vi "test comm.vi"() -> ()   [LabVIEW 2010]
uses:
  <userlib>/TIO Library 2010/TIO Stream Write.vi
  <userlib>/TIO Library 2010/TIO RPC Form Request.vi
  <userlib>/TIO Library 2010/TIO SLIP Serial Write.vi
  <userlib>/TIO Library 2010/TIO Form Packet.vi
  <userlib>/TIO Library 2010/TIO SLIP Encode.vi
  <userlib>/TIO Library 2010/TIO Serial Checksum CRC32.vi
panel:
  in  "flush":bool
  in  "milliseconds to wait":u32=100
  out "appended array 2":cluster{dbl, "start":dbl, "u32":u32}[](array[cluster]) {"start" format="%#.3f"}
  in  "Enum":enum16{"straight", "dstream"}(ring)
  out "Payload at dtream":string
  out "dstream info":T1
  out "Payload at timebase":string
  out "Payload at pstream":string
  out "pstreams out":T2(array[cluster])
  out "timebases out":T3(array[cluster])
  out "Payload at type 5":string
  out "appended array":u16[](array[numeric])
  in  "TIO State":T4={"Awaiting REP"=FALSE, "REQ ID"=500, "dstreams in"=[{"id"=0, "timebase id"=1, "period"=16, "offset"=0, "sample number"=10656, "total components"=6, "flags"=1, "components"=[{"pstream id"=0, "flags"=0, "period"=1, "offset"=0}, {"pstream id"=1, "flags"=1, "period"=1, "offset"=0}, {"pstream id"=32770, "flags"=0, "period"=8, "offset"=0}, {"pstream id"=32772, "flags"=0, "period"=8, "offset"=0}, {"pstream id"=32774, "flags"=1, "period"=64, "offset"=0}, {"pstream id"=2, "flags"=1, "period"=64, "offset"=0}]}, {"id"=0, "timebase id"=0, "period"=0, "offset"=0, "sample number"=0, "total components"=0, "flags"=0, "components"=[]}, {"id"=0, "timebase id"=0, "period"=0, "offset"=0, "sample number"=0, "total components"=0, "flags"=0, "components"=[]}, {"id"=0, "timebase id"=0, "period"=0, "offset"=0, "sample number"=0, "total components"=0, "flags"=0, "components"=[]}, {"id"=0, "timebase id"=0, "period"=0, "offset"=0, "sample number"=0, "total components"=0, "flags"=0, "components"=[]}, {"id"=0, "timebase id"=0, "period"=0, "offset"=0, "sample number"=0, "total components"=0, "flags"=0, "components"=[]}, {"id"=0, "timebase id"=0, "period"=0, "offset"=0, "sample number"=0, "total components"=0, "flags"=0, "components"=[]}, {"id"=0, "timebase id"=0, "period"=0, "offset"=0, "sample number"=0, "total components"=0, "flags"=0, "components"=[]}, {"id"=0, "timebase id"=0, "period"=0, "offset"=0, "sample number"=0, "total components"=0, "flags"=0, "components"=[]}, {"id"=0, "timebase id"=0, "period"=0, "offset"=0, "sample number"=0, "total components"=0, "flags"=0, "components"=[]}, {"id"=0, "timebase id"=0, "period"=0, "offset"=0, "sample number"=0, "total components"=0, "flags"=0, "components"=[]}, {"id"=0, "timebase id"=0, "period"=0, "offset"=0, "sample number"=0, "total components"=0, "flags"=0, "components"=[]}, {"id"=0, "timebase id"=0, "period"=0, "offset"=0, "sample number"=0, "total components"=0, "flags"=0, "components"=[]}, {"id"=0, "timebase id"=0, "period"=0, "offset"=0, "sample number"=0, "total components"=0, "flags"=0, "components"=[]}, {"id"=0, "timebase id"=0, "period"=0, "offset"=0, "sample number"=0, "total components"=0, "flags"=0, "components"=[]}, {"id"=0, "timebase id"=0, "period"=0, "offset"=0, "sample number"=0, "total components"=0, "flags"=0, "components"=[]}, {"id"=0, "timebase id"=0, "period"=0, "offset"=0, "sample number"=0, "total components"=0, "flags"=0, "components"=[]}, {"id"=0, "timebase id"=0, "period"=0, "offset"=0, "sample number"=0, "total components"=0, "flags"=0, "components"=[]}, {"id"=0, "timebase id"=0, "period"=0, "offset"=0, "sample number"=0, "total components"=0, "flags"=0, "components"=[]}, {"id"=0, "timebase id"=0, "period"=0, "offset"=0, "sample number"=0, "total components"=0, "flags"=0, "components"=[]}, {"id"=0, "timebase id"=0, "period"=0, "offset"=0, "sample number"=0, "total components"=0, "flags"=0, "components"=[]}, {"id"=0, "timebase id"=0, "period"=0, "offset"=0, "sample number"=0, "total components"=0, "flags"=0, "components"=[]}, {"id"=0, "timebase id"=0, "period"=0, "offset"=0, "sample number"=0, "total components"=0, "flags"=0, "components"=[]}, {"id"=0, "timebase id"=0, "period"=0, "offset"=0, "sample number"=0, "total components"=0, "flags"=0, "components"=[]}, {"id"=0, "timebase id"=0, "period"=0, "offset"=0, "sample number"=0, "total components"=0, "flags"=0, "components"=[]}, {"id"=0, "timebase id"=0, "period"=0, "offset"=0, "sample number"=0, "total components"=0, "flags"=0, "components"=[]}, {"id"=0, "timebase id"=0, "period"=0, "offset"=0, "sample number"=0, "total components"=0, "flags"=0, "components"=[]}, {"id"=0, "timebase id"=0, "period"=0, "offset"=0, "sample number"=0, "total components"=0, "flags"=0, "components"=[]}, {"id"=0, "timebase id"=0, "period"=0, "offset"=0, "sample number"=0, "total components"=0, "flags"=0, "components"=[]}, {"id"=0, "timebase id"=0, "period"=0, "offset"=0, "sample number"=0, "total components"=0, "flags"=0, "components"=[]}, {"id"=0, "timebase id"=0, "period"=0, "offset"=0, "sample number"=0, "total components"=0, "flags"=0, "components"=[]}, {"id"=0, "timebase id"=0, "period"=0, "offset"=0, "sample number"=0, "total components"=0, "flags"=0, "components"=[]}], "pstreams"=[{"id"=0, "timebase_id"=1, "period"=8, "offset"=0, "fmt"=-1, "flags"=0, "channels"=1, "type"=66, "name"="field", "column names"=["B"], "title"="Magnetic field", "units"="nT"}, {"id"=1, "timebase_id"=0, "period"=1, "offset"=0, "fmt"=-1, "flags"=0, "channels"=1, "type"=16, "name"="signal", "column names"=[""], "title"="Signal", "units"=""}, {"id"=2, "timebase_id"=0, "period"=1, "offset"=0, "fmt"=-1, "flags"=0, "channels"=1, "type"=16, "name"="status", "column names"=[""], "title"="Status", "units"=""}, {"id"=0, "timebase_id"=0, "period"=0, "offset"=0, "fmt"=0, "flags"=0, "channels"=0, "type"=0, "name"="", "column names"=[], "title"="", "units"=""}, {"id"=0, "timebase_id"=0, "period"=0, "offset"=0, "fmt"=0, "flags"=0, "channels"=0, "type"=0, "name"="", "column names"=[], "title"="", "units"=""}, {"id"=0, "timebase_id"=0, "period"=0, "offset"=0, "fmt"=0, "flags"=0, "channels"=0, "type"=0, "name"="", "column names"=[], "title"="", "units"=""}, {"id"=0, "timebase_id"=0, "period"=0, "offset"=0, "fmt"=0, "flags"=0, "channels"=0, "type"=0, "name"="", "column names"=[], "title"="", "units"=""}, {"id"=0, "timebase_id"=0, "period"=0, "offset"=0, "fmt"=0, "flags"=0, "channels"=0, "type"=0, "name"="", "column names"=[], "title"="", "units"=""}, {"id"=0, "timebase_id"=0, "period"=0, "offset"=0, "fmt"=0, "flags"=0, "channels"=0, "type"=0, "name"="", "column names"=[], "title"="", "units"=""}, {"id"=0, "timebase_id"=0, "period"=0, "offset"=0, "fmt"=0, "flags"=0, "channels"=0, "type"=0, "name"="", "column names"=[], "title"="", "units"=""}, {"id"=0, "timebase_id"=0, "period"=0, "offset"=0, "fmt"=0, "flags"=0, "channels"=0, "type"=0, "name"="", "column names"=[], "title"="", "units"=""}, {"id"=0, "timebase_id"=0, "period"=0, "offset"=0, "fmt"=0, "flags"=0, "channels"=0, "type"=0, "name"="", "column names"=[], "title"="", "units"=""}, {"id"=0, "timebase_id"=0, "period"=0, "offset"=0, "fmt"=0, "flags"=0, "channels"=0, "type"=0, "name"="", "column names"=[], "title"="", "units"=""}, {"id"=0, "timebase_id"=0, "period"=0, "offset"=0, "fmt"=0, "flags"=0, "channels"=0, "type"=0, "name"="", "column names"=[], "title"="", "units"=""}, {"id"=0, "timebase_id"=0, "period"=0, "offset"=0, "fmt"=0, "flags"=0, "channels"=0, "type"=0, "name"="", "column names"=[], "title"="", "units"=""}, {"id"=0, "timebase_id"=0, "period"=0, "offset"=0, "fmt"=0, "flags"=0, "channels"=0, "type"=0, "name"="", "column names"=[], "title"="", "units"=""}, {"id"=32768, "timebase_id"=1, "period"=8, "offset"=0, "fmt"=-1, "flags"=0, "channels"=1, "type"=66, "name"="_field.raw", "column names"=["B"], "title"="Magnetic field", "units"="nT"}, {"id"=32769, "timebase_id"=1, "period"=8, "offset"=0, "fmt"=-1, "flags"=0, "channels"=3, "type"=66, "name"="_spin.raw", "column names"=["measure", "reference", "output"], "title"="Spin lock", "units"=""}, {"id"=32770, "timebase_id"=1, "period"=8, "offset"=0, "fmt"=-1, "flags"=0, "channels"=3, "type"=66, "name"="spin", "column names"=["measure", "reference", "output"], "title"="Spin lock", "units"=""}, {"id"=32771, "timebase_id"=1, "period"=2, "offset"=0, "fmt"=-1, "flags"=0, "channels"=3, "type"=66, "name"="_laser.raw", "column names"=["measure", "reference", "output"], "title"="Laser lock", "units"=""}, {"id"=32772, "timebase_id"=1, "period"=2, "offset"=0, "fmt"=-1, "flags"=0, "channels"=3, "type"=66, "name"="laser", "column names"=["measure", "reference", "output"], "title"="Laser lock", "units"=""}, {"id"=32773, "timebase_id"=2, "period"=1, "offset"=0, "fmt"=-1, "flags"=0, "channels"=3, "type"=66, "name"="_therm.raw", "column names"=["measure", "reference", "output"], "title"="Cell temperature", "units"="°C"}, {"id"=32774, "timebase_id"=2, "period"=1, "offset"=0, "fmt"=-1, "flags"=0, "channels"=3, "type"=66, "name"="therm", "column names"=["measure", "reference", "output"], "title"="Cell temperature", "units"="°C"}, {"id"=32775, "timebase_id"=0, "period"=1, "offset"=0, "fmt"=-1, "flags"=0, "channels"=1, "type"=66, "name"="_cpu.raw", "column names"=[""], "title"="CPU load", "units"="%"}, {"id"=32776, "timebase_id"=0, "period"=1, "offset"=0, "fmt"=-1, "flags"=0, "channels"=1, "type"=66, "name"="cpu", "column names"=[""], "title"="CPU load", "units"="%"}, {"id"=0, "timebase_id"=0, "period"=0, "offset"=0, "fmt"=0, "flags"=0, "channels"=0, "type"=0, "name"="", "column names"=[], "title"="", "units"=""}, {"id"=0, "timebase_id"=0, "period"=0, "offset"=0, "fmt"=0, "flags"=0, "channels"=0, "type"=0, "name"="", "column names"=[], "title"="", "units"=""}, {"id"=0, "timebase_id"=0, "period"=0, "offset"=0, "fmt"=0, "flags"=0, "channels"=0, "type"=0, "name"="", "column names"=[], "title"="", "units"=""}, {"id"=0, "timebase_id"=0, "period"=0, "offset"=0, "fmt"=0, "flags"=0, "channels"=0, "type"=0, "name"="", "column names"=[], "title"="", "units"=""}, {"id"=0, "timebase_id"=0, "period"=0, "offset"=0, "fmt"=0, "flags"=0, "channels"=0, "type"=0, "name"="", "column names"=[], "title"="", "units"=""}, {"id"=0, "timebase_id"=0, "period"=0, "offset"=0, "fmt"=0, "flags"=0, "channels"=0, "type"=0, "name"="", "column names"=[], "title"="", "units"=""}, {"id"=0, "timebase_id"=0, "period"=0, "offset"=0, "fmt"=0, "flags"=0, "channels"=0, "type"=0, "name"="", "column names"=[], "title"="", "units"=""}], "timebases"=[{"id"=0, "source"=513, "epoch"=0, "start time"=0, "period numerator (µs)"=100000000, "period denominator (µs)"=1000, "flags"=0, "stability"=1, "source id"="\u0000\u0000\u0000\u0000\u0000À\u0001\u0000\u0000\u0000@\u0000\u001f\u0000\u0011P6W462 "}, {"id"=1, "source"=513, "epoch"=187833658, "start time"=0, "period numerator (µs)"=312500, "period denominator (µs)"=1000, "flags"=0, "stability"=1, "source id"="\u0000\u0000\u0000¬Å'7\u0001\u0000\u0000\u0000@\u0000\u001f\u0000\u0011P6W462 "}, {"id"=2, "source"=513, "epoch"=62622070, "start time"=0, "period numerator (µs)"=125000000, "period denominator (µs)"=1000, "flags"=0, "stability"=1, "source id"="\u0000\u0000\u0000\nף;\u0001\u0000\u0000\u0000@\u0000\u001f\u0000\u0011P6W462 "}, {"id"=0, "source"=0, "epoch"=0, "start time"=0, "period numerator (µs)"=0, "period denominator (µs)"=0, "flags"=0, "stability"=0, "source id"=""}, {"id"=0, "source"=0, "epoch"=0, "start time"=0, "period numerator (µs)"=0, "period denominator (µs)"=0, "flags"=0, "stability"=0, "source id"=""}, {"id"=0, "source"=0, "epoch"=0, "start time"=0, "period numerator (µs)"=0, "period denominator (µs)"=0, "flags"=0, "stability"=0, "source id"=""}, {"id"=0, "source"=0, "epoch"=0, "start time"=0, "period numerator (µs)"=0, "period denominator (µs)"=0, "flags"=0, "stability"=0, "source id"=""}, {"id"=0, "source"=0, "epoch"=0, "start time"=0, "period numerator (µs)"=0, "period denominator (µs)"=0, "flags"=0, "stability"=0, "source id"=""}, {"id"=0, "source"=0, "epoch"=0, "start time"=0, "period numerator (µs)"=0, "period denominator (µs)"=0, "flags"=0, "stability"=0, "source id"=""}, {"id"=0, "source"=0, "epoch"=0, "start time"=0, "period numerator (µs)"=0, "period denominator (µs)"=0, "flags"=0, "stability"=0, "source id"=""}, {"id"=0, "source"=0, "epoch"=0, "start time"=0, "period numerator (µs)"=0, "period denominator (µs)"=0, "flags"=0, "stability"=0, "source id"=""}, {"id"=0, "source"=0, "epoch"=0, "start time"=0, "period numerator (µs)"=0, "period denominator (µs)"=0, "flags"=0, "stability"=0, "source id"=""}, {"id"=0, "source"=0, "epoch"=0, "start time"=0, "period numerator (µs)"=0, "period denominator (µs)"=0, "flags"=0, "stability"=0, "source id"=""}, {"id"=0, "source"=0, "epoch"=0, "start time"=0, "period numerator (µs)"=0, "period denominator (µs)"=0, "flags"=0, "stability"=0, "source id"=""}, {"id"=0, "source"=0, "epoch"=0, "start time"=0, "period numerator (µs)"=0, "period denominator (µs)"=0, "flags"=0, "stability"=0, "source id"=""}, {"id"=0, "source"=0, "epoch"=0, "start time"=0, "period numerator (µs)"=0, "period denominator (µs)"=0, "flags"=0, "stability"=0, "source id"=""}, {"id"=0, "source"=0, "epoch"=0, "start time"=0, "period numerator (µs)"=0, "period denominator (µs)"=0, "flags"=0, "stability"=0, "source id"=""}, {"id"=0, "source"=0, "epoch"=0, "start time"=0, "period numerator (µs)"=0, "period denominator (µs)"=0, "flags"=0, "stability"=0, "source id"=""}, {"id"=0, "source"=0, "epoch"=0, "start time"=0, "period numerator (µs)"=0, "period denominator (µs)"=0, "flags"=0, "stability"=0, "source id"=""}, {"id"=0, "source"=0, "epoch"=0, "start time"=0, "period numerator (µs)"=0, "period denominator (µs)"=0, "flags"=0, "stability"=0, "source id"=""}, {"id"=0, "source"=0, "epoch"=0, "start time"=0, "period numerator (µs)"=0, "period denominator (µs)"=0, "flags"=0, "stability"=0, "source id"=""}, {"id"=0, "source"=0, "epoch"=0, "start time"=0, "period numerator (µs)"=0, "period denominator (µs)"=0, "flags"=0, "stability"=0, "source id"=""}, {"id"=0, "source"=0, "epoch"=0, "start time"=0, "period numerator (µs)"=0, "period denominator (µs)"=0, "flags"=0, "stability"=0, "source id"=""}, {"id"=0, "source"=0, "epoch"=0, "start time"=0, "period numerator (µs)"=0, "period denominator (µs)"=0, "flags"=0, "stability"=0, "source id"=""}, {"id"=0, "source"=0, "epoch"=0, "start time"=0, "period numerator (µs)"=0, "period denominator (µs)"=0, "flags"=0, "stability"=0, "source id"=""}, {"id"=0, "source"=0, "epoch"=0, "start time"=0, "period numerator (µs)"=0, "period denominator (µs)"=0, "flags"=0, "stability"=0, "source id"=""}, {"id"=0, "source"=0, "epoch"=0, "start time"=0, "period numerator (µs)"=0, "period denominator (µs)"=0, "flags"=0, "stability"=0, "source id"=""}, {"id"=0, "source"=0, "epoch"=0, "start time"=0, "period numerator (µs)"=0, "period denominator (µs)"=0, "flags"=0, "stability"=0, "source id"=""}, {"id"=0, "source"=0, "epoch"=0, "start time"=0, "period numerator (µs)"=0, "period denominator (µs)"=0, "flags"=0, "stability"=0, "source id"=""}, {"id"=0, "source"=0, "epoch"=0, "start time"=0, "period numerator (µs)"=0, "period denominator (µs)"=0, "flags"=0, "stability"=0, "source id"=""}, {"id"=0, "source"=0, "epoch"=0, "start time"=0, "period numerator (µs)"=0, "period denominator (µs)"=0, "flags"=0, "stability"=0, "source id"=""}, {"id"=0, "source"=0, "epoch"=0, "start time"=0, "period numerator (µs)"=0, "period denominator (µs)"=0, "flags"=0, "stability"=0, "source id"=""}]}
  out "Data Out":T5(array[cluster])=[{"Name"="gmr", "Waveform"={"start"=0.0, "dt"=1.0, "Timeseries"=[[-1045203.625, 2103369.25, -524451.0625]]}}, {"Name"="accel", "Waveform"={"start"=0.0, "dt"=1.0, "Timeseries"=[[0.4673272967338562, -9.214466094970703, -3.09728741645813]]}}, {"Name"="gyro", "Waveform"={"start"=0.0, "dt"=1.0, "Timeseries"=[[0.019417261704802513, 0.00881516095250845, 0.006293708924204111]]}}, {"Name"="bar", "Waveform"={"start"=0.0, "dt"=1.0, "Timeseries"=[[0.0]]}}, {"Name"="therm", "Waveform"={"start"=0.0, "dt"=1.0, "Timeseries"=[[0.0]]}}] {"Waveform"."start" format="%#.3f"}
  out "output cluster":cluster{u16, "u32":u32, string}
  in  "Payload In":string
  out "Type":u16(ring)=2 items=["Invalid", "Log", "RPC Request", "RPC Reply", "RPC Error", "Stream Description", "User"]
  in  "read cont":bool
  out "sent Request ID":u16=60741 format="%0d"
  out "Request ID":u16
  out "Parsed Payload":string
  out "TC Connection":T6={"Type"=enum."Serial", "URL"="serial:///dev/cu.usbserial-00000", "TO"=500, "Addr"=0, "Port"=0, "TCP"=refnum, "UDP"=refnum, "Route"=""}
  out "Routing Matches":bool
  out "length":i32
  out "Connected":bool
  in  "Topic":string
  in  "stop":bool
  out "Payload":string
  out "error out":errorcluster
  in  "read":bool
  in  "send":bool
  in  "URL":refnum<visa-resource-name>="tcp://localhost"
  out "ID":string="Twinleaf VM4 R4"
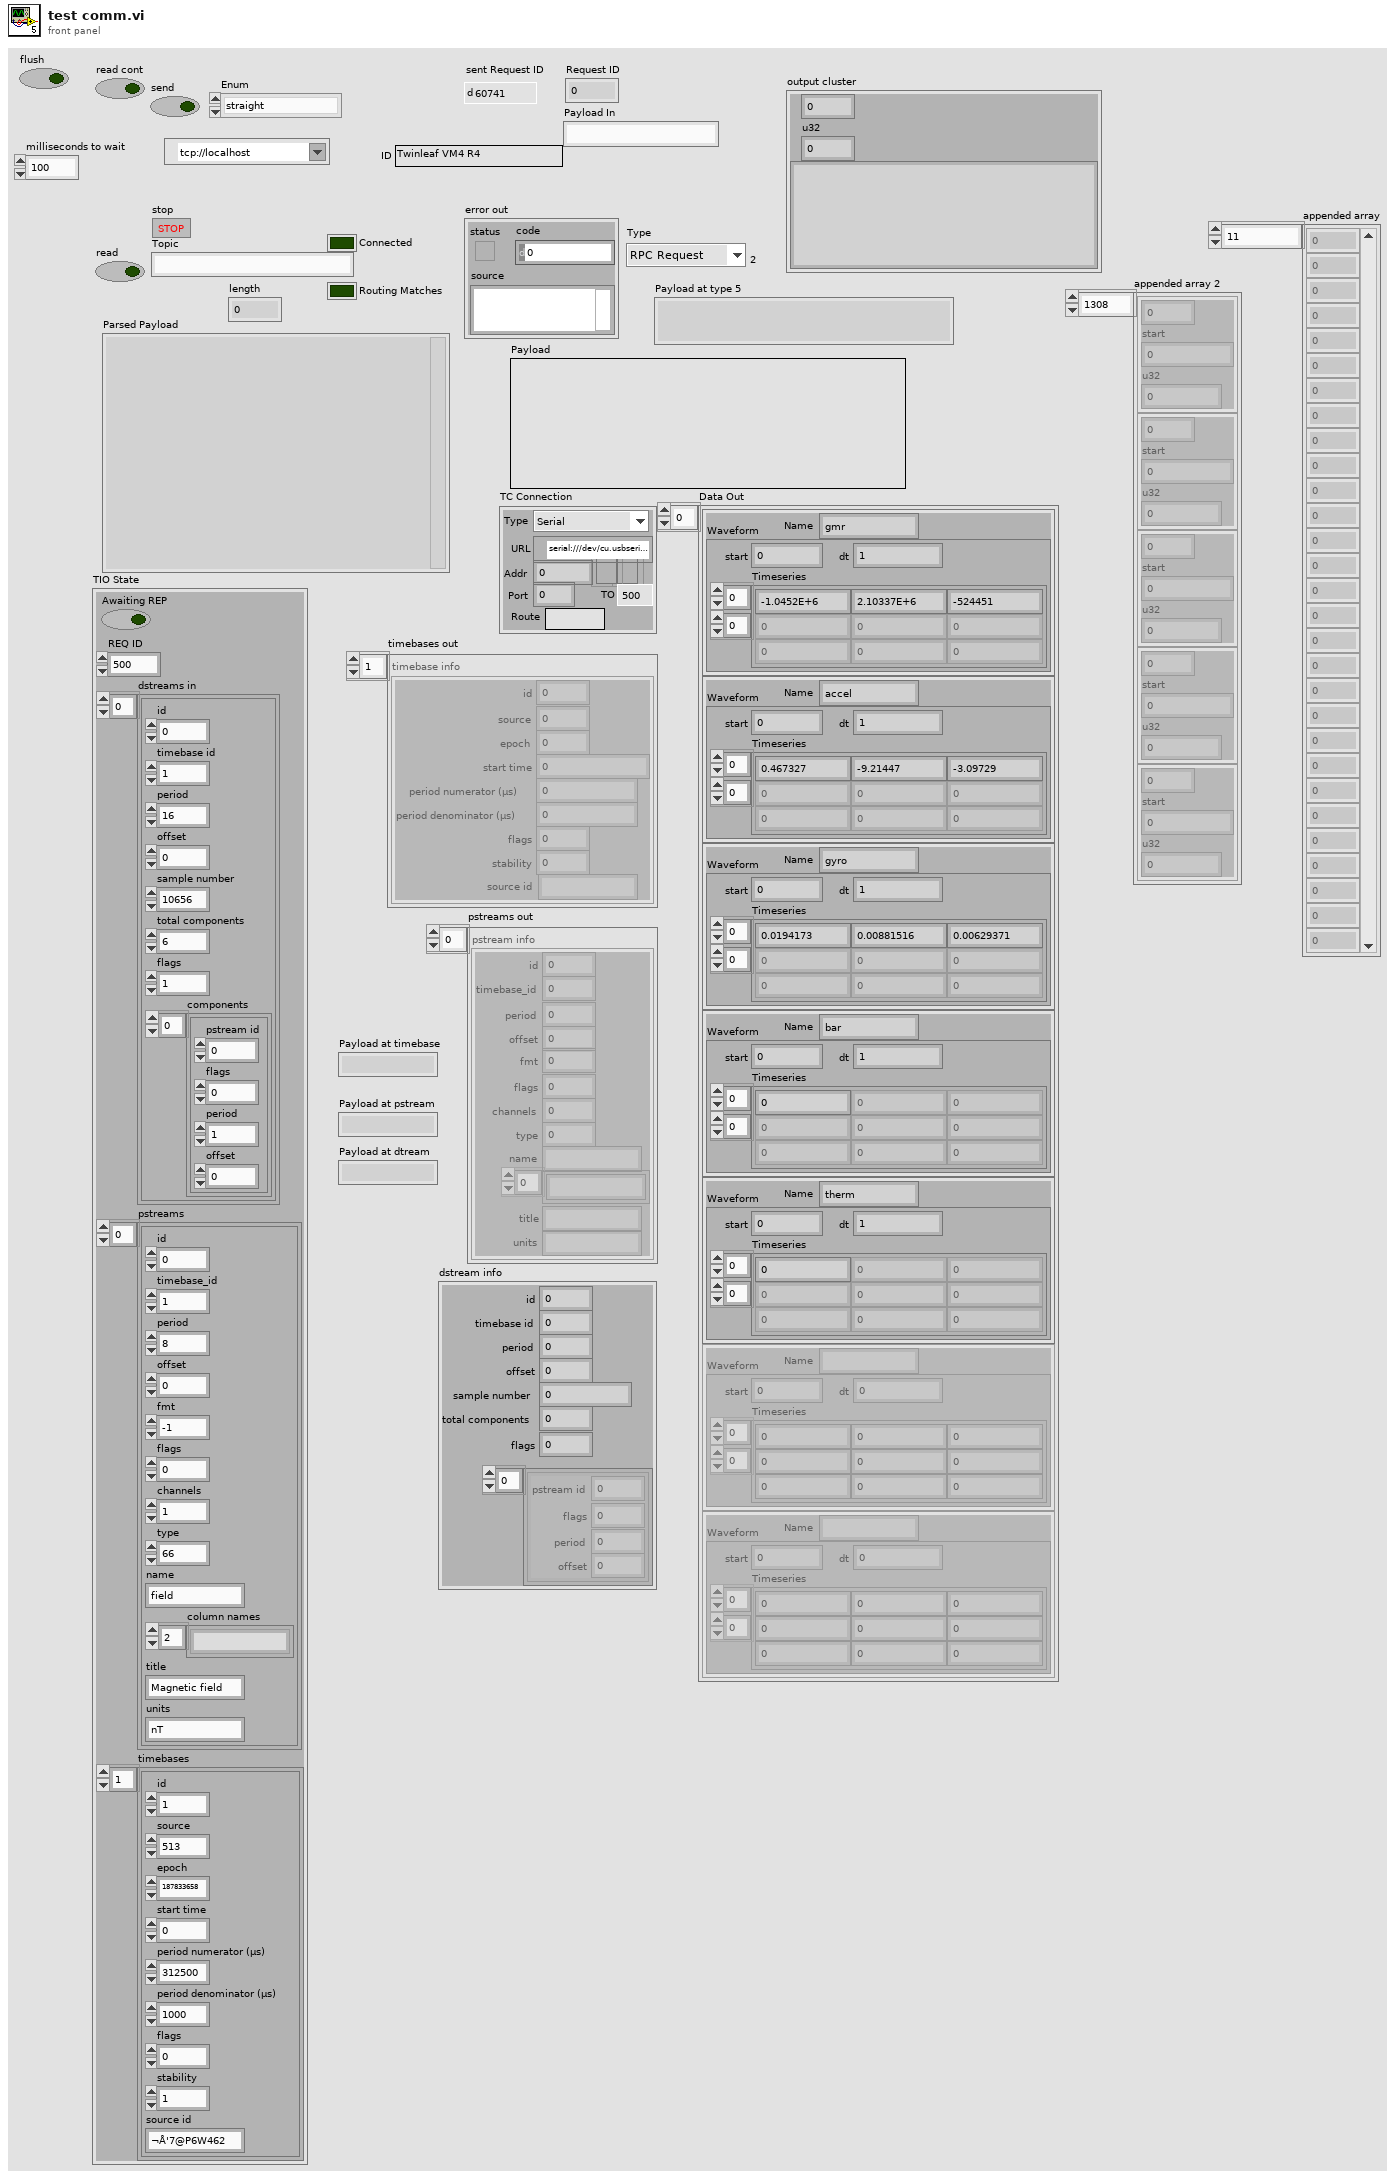
[diagram p1: front panel]
types:
  T1 = cluster{"id":u16, "timebase id":u16, "period":u32, "offset":u32, "sample number":u64, "total components":u16, "flags":u16, cluster{"pstream id":u16, "flags":u16, "period":u32, "offset":u32}[]}
  T2 = cluster{"id":u16, "timebase_id":u16, "period":u32, "offset":u32, "fmt":i32, "flags":u16, "channels":u16, "type":u8, "name":string, string[], "title":string, "units":string}[]
  T3 = cluster{"id":u16, "source":u8, "epoch":u8, "start time":u64, "period numerator (µs)":u32, "period denominator (µs)":u32, "flags":u32, "stability":sgl, "source id":string}[]
  T4 = cluster{"Awaiting REP":bool, "REQ ID":u32, "dstreams in":cluster{"id":u16, "timebase id":u16, "period":u32, "offset":u32, "sample number":u64, "total components":u16, "flags":u16, "components":cluster{"pstream id":u16, "flags":u16, "period":u32, "offset":u32}[]}[], "pstreams":cluster{"id":u16, "timebase_id":u16, "period":u32, "offset":u32, "fmt":i32, "flags":u16, "channels":u16, "type":u8, "name":string, "column names":string[], "title":string, "units":string}[], "timebases":cluster{"id":u16, "source":u16, "epoch":u32, "start time":u32, "period numerator (µs)":i32, "period denominator (µs)":u16, "flags":u16, "stability":u8, "source id":string}[]}
  T5 = cluster{"Name":string, "Waveform":cluster{"start":dbl, "dt":dbl, "Timeseries":dbl[][]}}[]
  T6 = cluster{"Type":enum16{"Serial", "TCP", "UDP", "mUDP"}, "URL":refnum<visa-resource-name>, "TO":u32, "Addr":u32, "Port":i32, "TCP":refnum<k5>, "UDP":refnum<k16>, "Route":string}
  T7 = enum16{"big-endian, network order", "native, host order", "little-endian"}
  T8 = cluster{"Name":string, "Waveform":cluster{"start":dbl, "dt":dbl, "Timeseries":dbl[][]}}
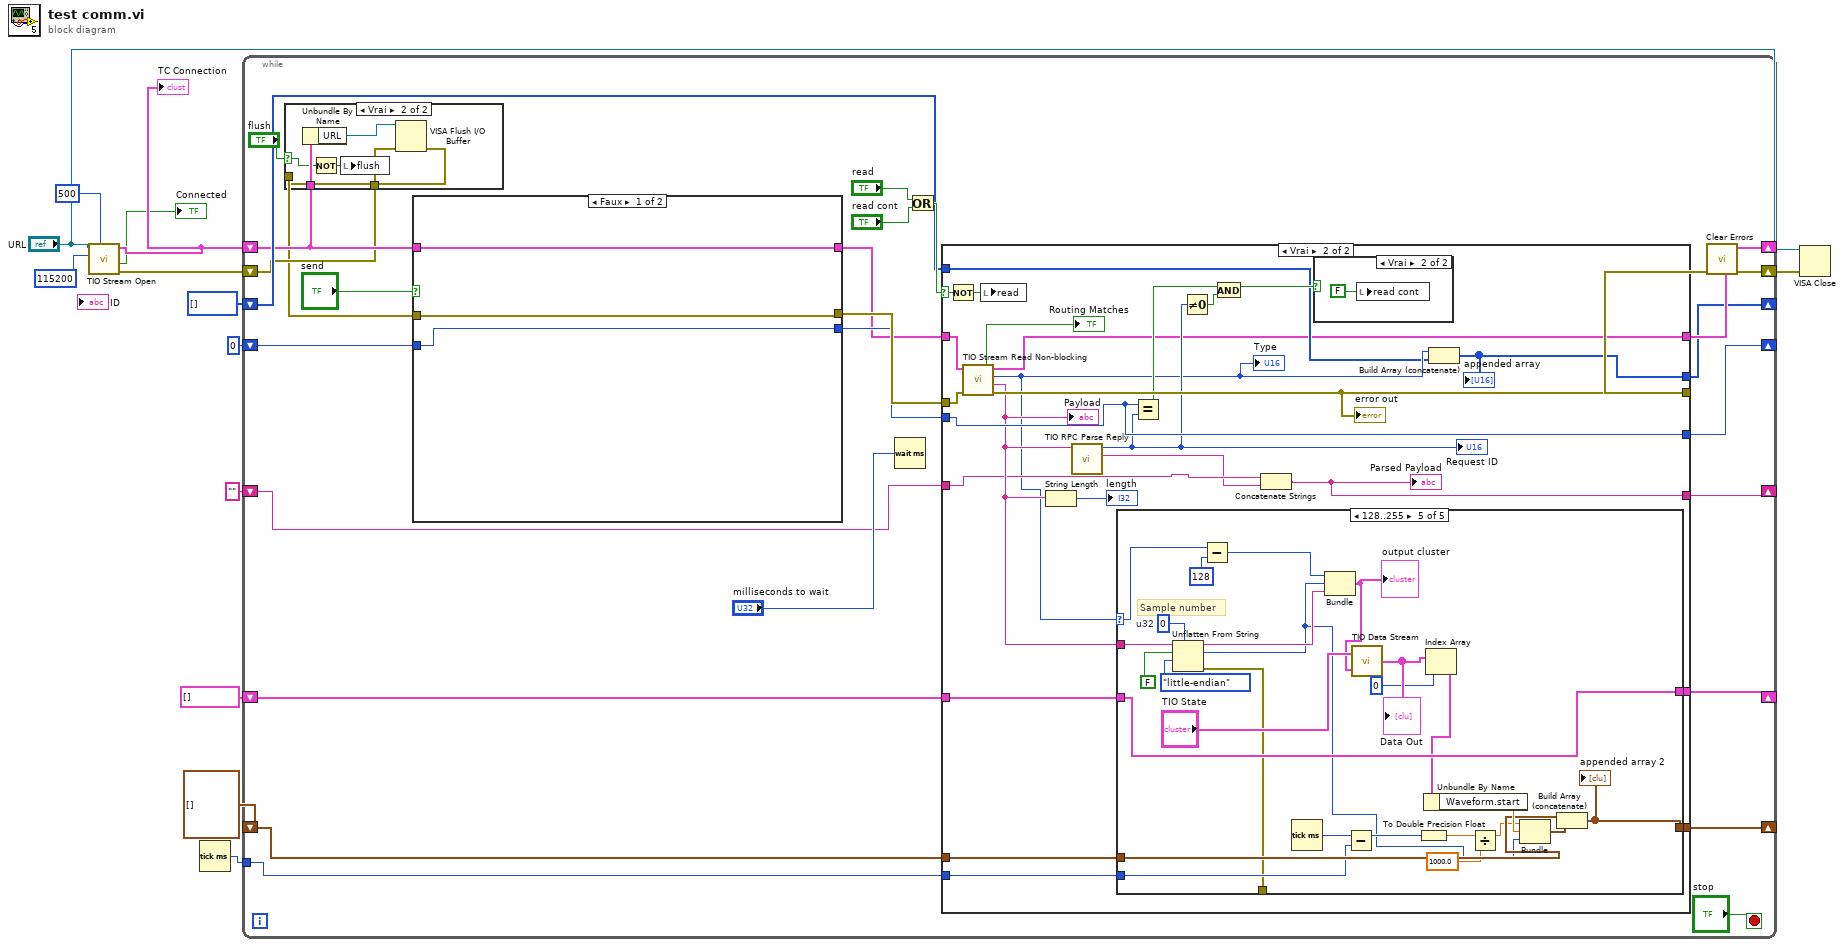
[diagram p0: block diagram]
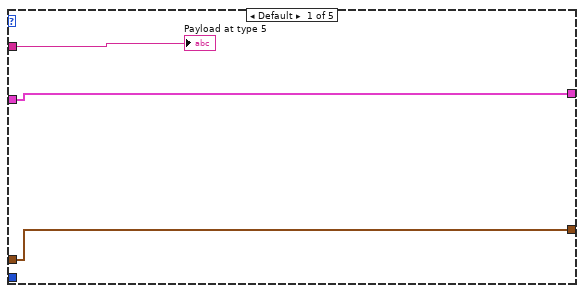
[diagram p4: hidden frame]
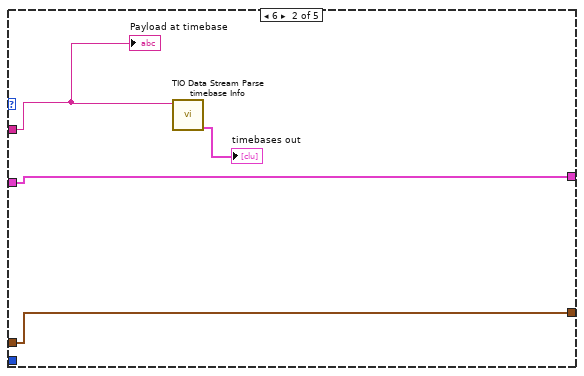
[diagram p5: hidden frame]
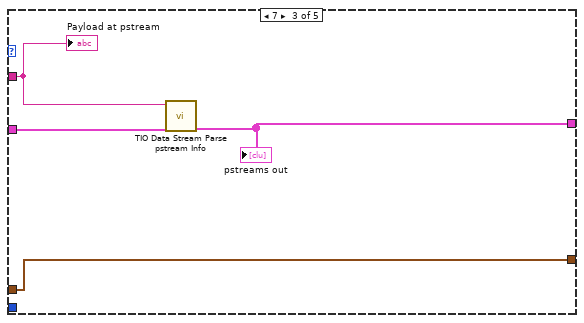
[diagram p6: hidden frame]
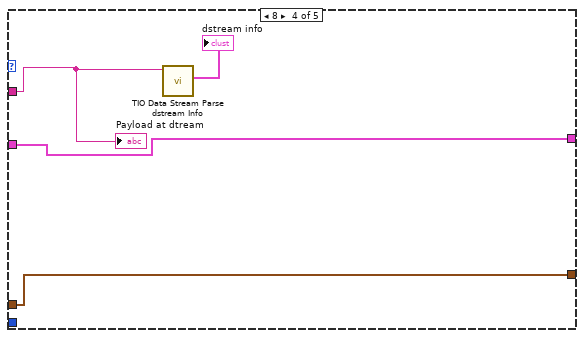
[diagram p7: hidden frame]
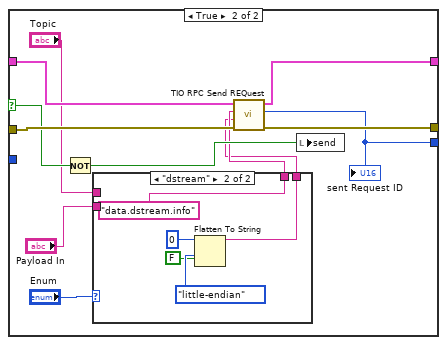
[diagram p9: hidden frame]
diagram:
  n1 = call <userlib>:"TIO Stream Open.vi"("Port timeout"=u32 500, "Default baud"=u32 115200, "URL"="URL") -> ("error out"=w10:errorcluster, "Connected"=→"Connected":bool, "TC Connection"=w13:T6)  [unwired: 6 in]
  "TC Connection" <- w13
  n2 = Tick Count (ms)() -> (millisecond timer value=w3:u32)
  n3 = while {
    shift-right: [w37] -> _
    shift-left: w13 -> [w17]
    shift-right: [w35] -> w12
    shift-left: w10 -> [w16]
    shift-right: [w31] -> _
    shift-left: u16 0 ("Request ID") -> [w30]
    shift-right: [w27] -> _
    shift-left: "" ("Payload") -> [w26]
    shift-right: [w25] -> _
    shift-left: u16[] [] -> [w24]
    shift-right: [w22] -> _
    shift-left: T2 [] ("pstreams out") -> [w21]
    shift-right: [w20] -> _
    shift-left: cluster{dbl, "start":dbl, "u32":u32}[] [] -> [w19]
    tunnel: w3 -> [w18]
    stop <- "stop" stop-if-true
    n4 = case shown="Vrai" "flush" {
      selector: "flush" -> [_ w42]
      tunnel: w17 -> [_ w47]
      tunnel: w16 -> [w41 w45]
      tunnel: [w41 w44] -> w15
      frame False {
      }
      frame True {
        n5 = Unbundle By Name(w47) -> ("URL"=w46:refnum<visa-resource-name>)
        n6 = Not(x=w42) -> (.not. x?=w43:bool)
        n7 = local write "flush"(w43) -> ()
        n8 = VISA Flush I/O Buffer(VISA resource name=w46, error in (no error)=w45) -> (error out=w44:errorcluster)  [unwired: 1 in, 1 out]
      }
    }
    n9 = case shown="Faux" "send" {
      selector: "send" -> [_ w132]
      tunnel: w15 -> [w123 w136]
      tunnel: w17 -> [w124 w135]
      tunnel: [w124 w134] -> w23
      tunnel: [w123 w133] -> w39
      tunnel: [w122 w130] -> w32
      tunnel: w30 -> [w122 _]
      frame False {
      }
      frame True {
        n10 = Not(x=w132) -> (.not. x?=w131:bool)
        n11 = case shown="\"dstream\"" "Enum" {
          tunnel: "Topic" -> [w138 _]
          tunnel: "Payload In" -> [w137 _]
          tunnel: [w138 "data.dstream.info" ("Topic")] -> w126
          tunnel: [w137 w140] -> w125
          frame "straight", Default {
          }
          frame "dstream" {
            n12 = Flatten To String(anything=u16 0, prepend array or string size? (T)=FALSE, byte order (0:big-endian, network order)=T7."little-endian") -> (data string=w140:string)  [unwired: 1 in, 2 out]
          }
        }
        n13 = call <userlib>:"TIO RPC Send REQuest.vi"("error in (no error)"=w136, "Payload"=w125, "Topic"=w126, "TC Connection"=w135) -> ("error out"=w133:errorcluster, "Request ID"=w130:u16, "TC Connection"=w134:T6)  [unwired: 5 in]
        "sent Request ID" <- w130
        n14 = local write "send"(w131) -> ()
      }
    }
    n15 = Wait (ms)(milliseconds to wait="milliseconds to wait") -> ()  [unwired: 1 out]
    n16 = Or(x="read", y="read cont") -> (x .or. y?=w34:bool)
    n17 = case shown="Vrai" w34 {
      selector: w34 -> [_ w77]
      tunnel: w23 -> [w54 w56]
      tunnel: w39 -> [w53 w79]
      tunnel: [w54 w55] -> w37
      tunnel: [w53 w78] -> w28
      tunnel: w32 -> [w52 w73]
      tunnel: [w52 w73] -> w31
      tunnel: [w51 w65] -> w27
      tunnel: w26 -> [w51 w67]
      tunnel: [w50 w63] -> w25
      tunnel: w24 -> [w50 w62]
      tunnel: [w49 w61] -> w22
      tunnel: w21 -> [w49 w60]
      tunnel: [w48 w59] -> w20
      tunnel: w19 -> [w48 w58]
      tunnel: w18 -> [_ w57]
      frame False {
      }
      frame True {
        n18 = Not(x=w77) -> (.not. x?=w76:bool)
        n19 = call <userlib>:"TIO Stream Read Non-blocking.vi"("error in (no error)"=w79, "TC Connection"=w56) -> ("error out"=w78:errorcluster, "Payload"=w71:string, "Type"=w64:u16, "TC Connection"=w55:T6, "Routing Matches"=→"Routing Matches":bool)  [unwired: 4 in, 1 out]
        "Payload" <- w71
        "Type" <- w64
        "error out" <- w78
        n20 = local write "read"(w76) -> ()
        n21 = String Length(string=w71) -> (length=→"length":i32)
        n22 = call <userlib>:"TIO RPC Parse Reply.vi"("Payload"=w71) -> ("Payload"=w66:string, "Request ID"=w68:u16)  [unwired: 9 in]
        "Request ID" <- w68
        n23 = case shown="128..255" w64 {
          selector: w64 -> [_ _ _ _ w114]
          tunnel: w71 -> [w82 w86 w90 w94 w113]
          tunnel: [w81 w84 w89 w92 w110] -> w61
          tunnel: w60 -> [w81 w84 w88 w92 w110]
          tunnel: [w80 w83 w87 w91 w102] -> w59
          tunnel: w58 -> [w80 w83 w87 w91 w104]
          tunnel: w57 -> [_ _ _ _ w98]
          tunnel: [_ _ _ _ w95] -> _
          frame Default {
            "Payload at type 5" <- w82
          }
          frame 6 {
            n24 = call <userlib>:"TIO Data Stream Parse timebase Info.vi"("timebase info raw"=w86) -> ("timebases out"=→"timebases out":T3)  [unwired: 10 in]
            "Payload at timebase" <- w86
          }
          frame 7 {
            n25 = call <userlib>:"TIO Data Stream Parse pstream Info.vi"("pstreams in"=w88, "pstream info raw"=w90) -> ("pstreams out"=w89:T2)  [unwired: 9 in]
            "pstreams out" <- w89
            "Payload at pstream" <- w90
          }
          frame 8 {
            n26 = call <userlib>:"TIO Data Stream Parse dstream Info.vi"("dstream info raw"=w94) -> ("dstream info"=→"dstream info":T1)  [unwired: 9 in, 1 out]
            "Payload at dtream" <- w94
          }
          frame 128..255 {
            w116 = u32 0  # u32
            # "Sample number"
            n27 = Unflatten From String(type=w116, binary string=w113, data includes array or string size? (T)=FALSE, byte order (0:big-endian, network order)=T7."little-endian") -> (rest of the binary string=w115:string, value=w96:u32, error out=w95:errorcluster)  [unwired: 1 in]
            n28 = Subtract(x=w114, y=u16 128) -> (x-y=w119:u16)
            n29 = Tick Count (ms)() -> (millisecond timer value=w106:u32)
            n30 = Bundle(w119, "u32"=w96, w115) -> (w111:cluster{u16, "u32":u32, string})  [unwired: 1 in]
            "output cluster" <- w111
            n31 = Subtract(x=w106, y=w98) -> (x-y=w99:u32)
            n32 = call <userlib>:"TIO Data Stream.vi"("Raw Data"=w111, "TIO State"="TIO State") -> ("Data Out"=w109:T5)
            "Data Out" <- w109
            n33 = To Double Precision Float(number=w99) -> (double precision float=w97:dbl)
            n34 = Index Array(array=w109, index=0) -> (element=w107:T8)
            n35 = Unbundle By Name(w107) -> ("Waveform.start"=w105:dbl)
            n36 = Divide(x=w97, y=1000.0) -> (x/y=w101:dbl)
            n37 = Bundle(w101, "start"=w105, "u32"=w96) -> (w103:cluster{dbl, "start":dbl, "u32":u32})  [unwired: 1 in]
            n38 = Build Array (concatenate)(w104, w103) -> (w102:cluster{dbl, "start":dbl, "u32":u32}[])
            "appended array 2" <- w102
          }
        }
        n39 = Equal?(x=w73, y=w68) -> (x = y?=w72:bool)
        n40 = Not Equal To 0?(x=w68) -> (x != 0?=w69:bool)
        n41 = And(x=w72, y=w69) -> (x .and. y?=w70:bool)
        n42 = Concatenate Strings(w67, w66) -> (w65:string)
        "Parsed Payload" <- w65
        n43 = case shown="Vrai" w70 {
          frame False {
          }
          frame True {
            n44 = local write "read cont"(FALSE ("read cont")) -> ()
          }
        }
        n45 = Build Array (concatenate)(w64, w62) -> (w63:u16[])
        "appended array" <- w63
      }
    }
    n46 = call <vilib>:"Clear Errors.vi"("error in (no error)"=w28) -> ("error out"=w35:errorcluster)  [unwired: 6 in]
  }
  n47 = VISA Close(VISA resource name="URL", error in (no error)=w12) -> ()  [unwired: 1 out]
